vi "CAN BOOT Set Addr Offset.vi"(5 "TimeOutOfMs":u32, 6 "pBufferSize":u16, 7 "AddrOffset":u32, 9 "NAD":u8, 10 "CANIndex":i32, 11 "DevHandle":i32) -> (3 "function return":i32, 4 "pBufferSize out":u16)   [LabVIEW 2010, in "can_bootloader.lvlib"]
doc: "int WINAPI CAN_BOOT_SetAddrOffset(int DevHandle,int CANIndex,unsigned char NAD,unsigned int AddrOffset,unsigned short *pBufferSize,unsigned int TimeOutOfMs);"
uses:
  can_bootloader.lvlib
  USB2XXX/trunk/USB2XXX/USB2XXX/vs2010/Release/USB2XXX.dll
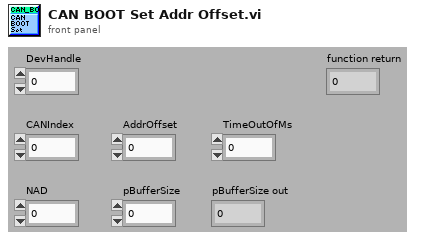
[diagram p1: front panel]
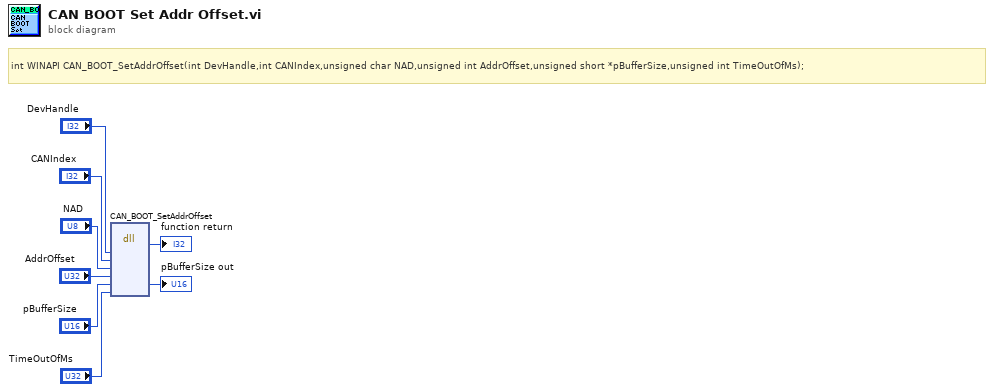
[diagram p0: block diagram]
diagram:
  # "int WINAPI CAN_BOOT_SetAddrOffset(int DevHandle,int CANIndex,unsigned char NAD,unsigned int AddrOffset,unsigned short *pBufferSize,unsigned int TimeOutOfMs);"
  n1 = dll-call lib="E:/OtherWork/STM32/USB2XXX/trunk/USB2XXX/USB2XXX/vs2010/Release/USB2XXX.*" fn="CAN_BOOT_SetAddrOffset"("DevHandle"="DevHandle", "CANIndex"="CANIndex", "NAD"="NAD", "AddrOffset"="AddrOffset", "pBufferSize"="pBufferSize", "TimeOutOfMs"="TimeOutOfMs") -> (→"function return":i32, "pBufferSize"=→"pBufferSize out":u16)  [unwired: 8 in, 2 out]
